vi "VOLTAJE_LECTURA.vi"() -> ()   [LabVIEW 2021]
uses:
  <vilib>/Instr/_visa.llb/Select Event Type.ctl
  <vilib>/Instr/_visa.llb/VISA Configure Serial Port (Instr).vi
panel:
  out "Volt IN":dbl
  out "Collected Signals":dynamicdata(graph)
  out "x/y":dbl
  out "read buffer":string
  in  "Event Type":T1=1073684491 items=["Service Request"=1073684491, "Trigger"=3221168138, "Clear"=1073684493, "VXI Signal"=1073684512, "VXI/VME Interrupt"=3221168161, "VXI/VME Sysfail"=1073684509, "VXI/VME Sysreset"=1073684510, "GPIB CIC"=1073684498, "GPIB Talk"=1073684499, "GPIB Listen"=1073684500, "PXI Interrupt"=1073684514, "Serial Break"=1073684515, "Serial TermChar"=1073684516, "Serial CTS"=1073684521, "Serial DSR"=1073684522, "Serial DCD"=1073684524, "Serial RI"=1073684526, "Serial Character"=1073684533, "USB Interrupt"=1073684535, "All Enabled"=1073709055]
  in  "VISA resource name":refnum<visa-resource-name>
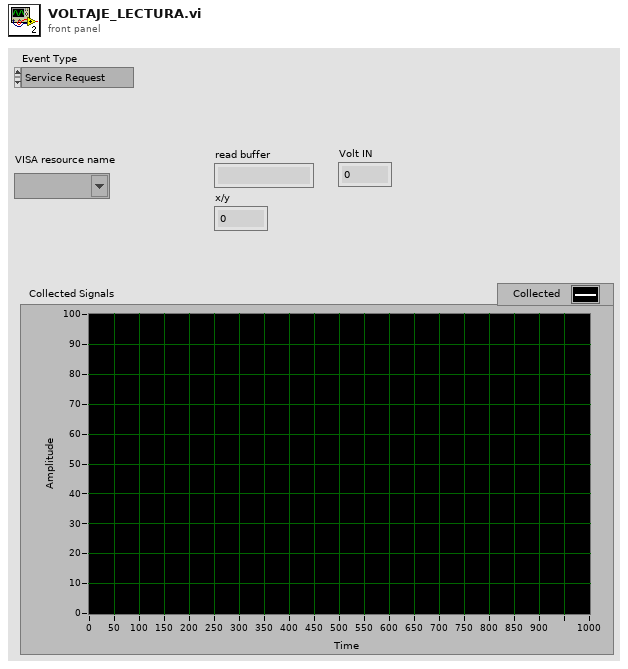
[diagram p1: front panel]
types:
  T1 = typedef "Select Event Type.ctl" = u32
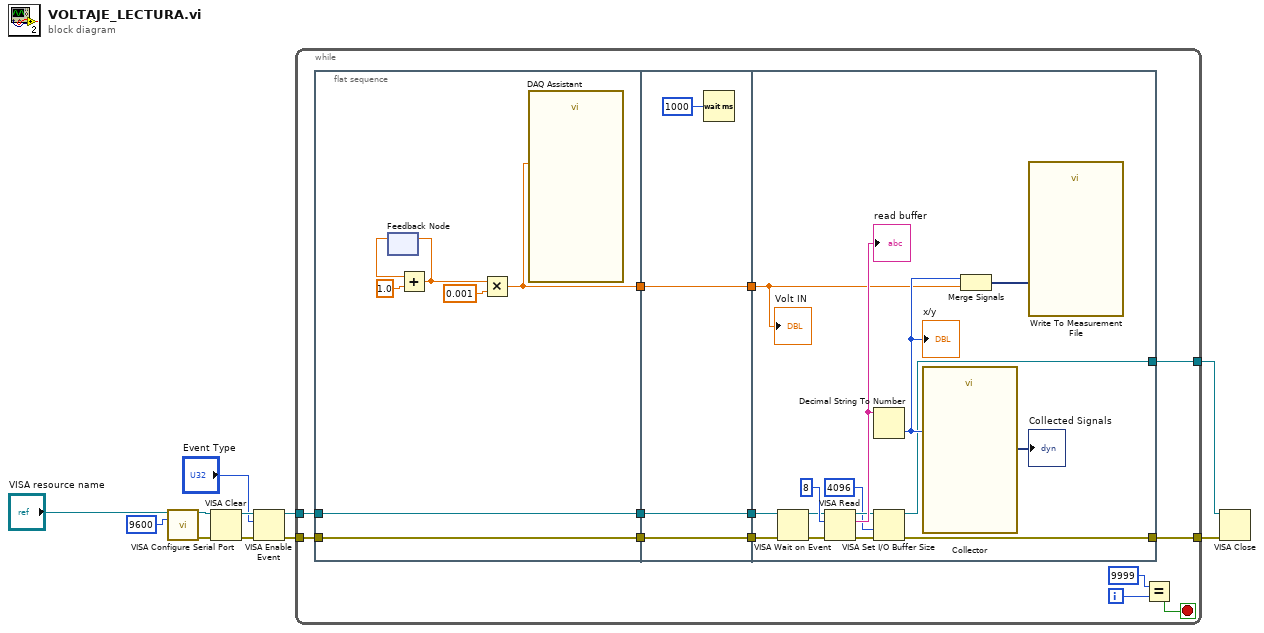
[diagram p0: block diagram]
diagram:
  n1 = call-poly "VISA Configure Serial Port"("VISA resource name"="VISA resource name", "baud rate (9600)"=u32 9600) -> ("VISA resource name out"=w9:refnum<visa-resource-name>, "error out"=w8:errorcluster)  [unwired: 12 in]
  n2 = VISA Clear(VISA resource name=w9, error in (no error)=w8) -> (VISA resource name out=w7:refnum<visa-resource-name>, error out=w6:errorcluster)
  n3 = VISA Enable Event(8:w6, 10:"Event Type", 11:w7) -> (0:w3:errorcluster, 3:w4:refnum<visa-resource-name>)  [unwired: 1 in]
  n4 = while {
    tunnel: w4 -> [w19]
    tunnel: w3 -> [w16]
    tunnel: [w15] -> w2
    tunnel: [w14] -> w1
    i -> [w24]
    stop <- w22 stop-if-true
    n5 = flat-sequence {
      tunnel: [w27] -> w20
      tunnel: w19 -> [w27]
      tunnel: [w26] -> w17
      tunnel: w16 -> [w26]
      tunnel: [w25] -> w13
      tunnel: [w34] -> w21
      tunnel: w20 -> [w34]
      tunnel: [w33] -> w18
      tunnel: w17 -> [w33]
      tunnel: w13 -> [w32]
      tunnel: [w32] -> w12
      tunnel: w21 -> [w42]
      tunnel: w18 -> [w41]
      tunnel: [w39] -> w15
      tunnel: [w38] -> w14
      tunnel: w12 -> [w36]
      frame #0 {
        n6 = feedback #1() -> (w30:dbl)  [unwired: 1 in]
        n7 = Add(x=w30, y=1.0) -> (x+y=w31:dbl)
        n8 = feedback-in #1(w31) -> ()
        n9 = Multiply(x=w31, y=0.001) -> (x*y=w25:dbl)
        n10 = call "DAQ Assistant"("data"=w25) -> ()  [unwired: 17 in, 2 out]
      }
      frame #1 {
        n11 = Wait (ms)(milliseconds to wait=u32 1000) -> ()  [unwired: 1 out]
      }
      frame #2 {
        n12 = VISA Wait on Event(8:w41, 11:w42) -> (0:w43:errorcluster, 3:w44:refnum<visa-resource-name>)  [unwired: 3 in, 2 out]
        n13 = VISA Read(VISA resource name=w44, byte count=u32 8, error in (no error)=w43) -> (VISA resource name out=w48:refnum<visa-resource-name>, read buffer=w50:string, error out=w47:errorcluster)  [unwired: 1 out]
        "read buffer" <- w50
        n14 = Decimal String To Number(string=w50) -> (number=w40:i32)  [unwired: 2 in, 1 out]
        "x/y" <- w40
        n15 = VISA Set I/O Buffer Size(VISA resource name=w48, size (4096)=u32 4096, error in (no error)=w47) -> (VISA resource name out=w39:refnum<visa-resource-name>, error out=w38:errorcluster)  [unwired: 1 in]
        n16 = call "Collector"("Signals"=w40) -> ("Collected Signals"=→"Collected Signals":dynamicdata)  [unwired: 9 in, 1 out]
        n17 = Merge Signals(w40, w36) -> (w37:dynamicdata)
        n18 = call "Write To Measurement File"("Signals"=w37) -> ()  [unwired: 16 in, 3 out]
        "Volt IN" <- w36
      }
    }
    n19 = Equal?(x=9999, y=w24) -> (x = y?=w22:bool)
  }
  n20 = VISA Close(VISA resource name=w2, error in (no error)=w1) -> ()  [unwired: 1 out]
